vi "LVClasse_SurfaceFloat Set Data.vi"(0 "SurfaceFloat in":refnum<class "SurfaceFloat.lvclass">, 5 "data":sgl[][](array[numeric]), 11 "error in (no error)":errorcluster) -> (4 "SurfaceFloat out":refnum<class "SurfaceFloat.lvclass">, 15 "error out":errorcluster)   [LabVIEW 2020, in "SurfaceFloat.lvclass"]
doc: "Get write access Surface buffer.\n\n--------------------------------------------------------------------------------\n\n<B>SurfaceIn </B> : Surface object.\n<B>SurfaceOut </B> : Surface object.\n<B>data </B> : Surface buffer to set.\n<B>ErrorIn </B> : Error\n<B>ErrorOut </B> : Error\n\n--------------------------------------------------------------------------------"
uses:
  SurfaceFloat.lvclass
  SurfaceFloat.lvclass/SurfaceFloat.ctl
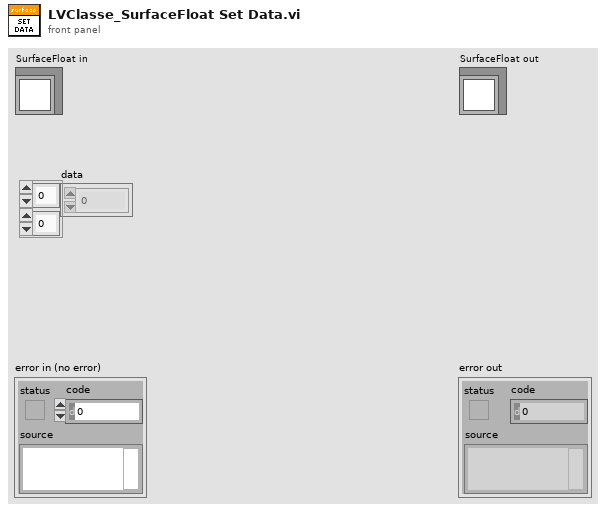
[diagram p1: front panel]
types:
  T1 = typedef "General dimensions definition.ctl" = cluster{"Size":T2, "Step":T3}
  T2 = typedef "Point2D.ctl" = cluster{"X":u32, "Y":u32}
  T3 = typedef "Point2Df.ctl" = cluster{"X":sgl, "Y":sgl}
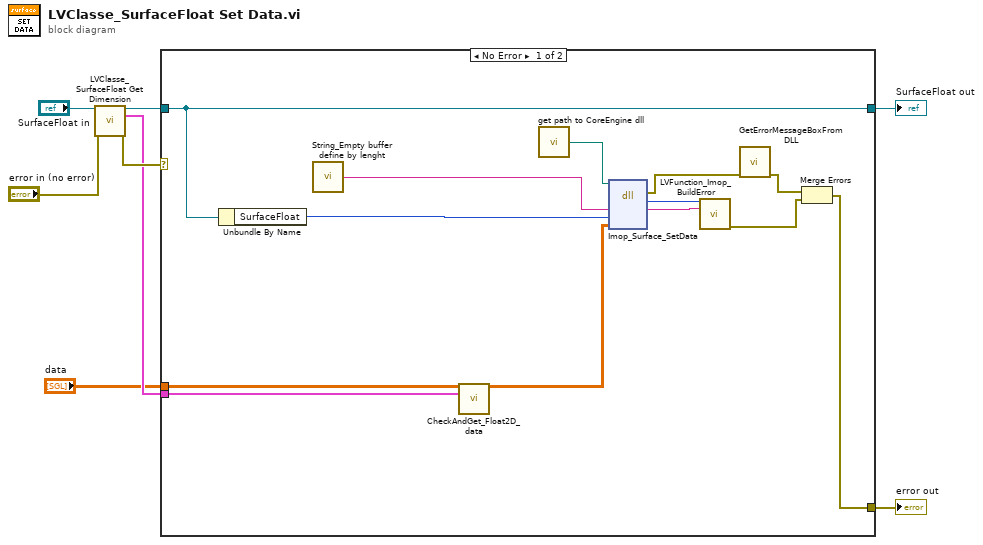
[diagram p0: block diagram]
diagram:
  n1 = call "LVClasse_SurfaceFloat Get Dimension.vi"("SurfaceFloat in"="SurfaceFloat in", "error in (no error)"="error in (no error)") -> ("SurfaceFloat out"=w3:refnum<class "SurfaceFloat.lvclass">, "Dimensions_um"=w2:T1, "error out"=w4:errorcluster)  [unwired: 11 in]
  n2 = case shown="No Error" w4 {
    selector: w4 -> [_ w23]
    tunnel: [w12 w23] -> w8
    tunnel: [w16 w22] -> w7
    tunnel: w3 -> [w16 w22]
    tunnel: w2 -> [w11 _]
    tunnel: "data" -> [w9 _]
    frame No Error {
      n3 = Unbundle By Name(w16) -> ("SurfaceFloat"=w15:i32)
      n4 = call "String_Empty buffer define by lenght.vi"() -> ("Empty buffer"=w19:string)  [unwired: 1 in]
      n5 = call "CheckAndGet_Float2D_data.vi"("data in"=w9, "Dimensions_um"=w11) -> ("data out"=w10:sgl[][])  [unwired: 13 in]
      n6 = call "get path to CoreEngine dll.vi"() -> ("path to c_interface_vc100.dll"=w18:path)  [unwired: 12 in, 3 out]
      n7 = dll-call lib="D:/2_trunk/Soft_haso/ImOpCoreEngine4_LV2011/DLLs/ImopEngine4_vc100.dll" fn="Imop_Surface_SetData"(path in=w18, "message"=w19, "surface"=w15, "data"=w10) -> (error out=w17:errorcluster, "return type"=w21:i32, "message"=w20:string)  [unwired: 4 in, 1 out]
      n8 = call "LVFunction_Imop_BuildError.vi"("code"=w21, "String to Prepend to source (\"\")"=w20) -> ("error out"=w13:errorcluster)  [unwired: 13 in]
      n9 = call "GetErrorMessageBoxFromDLL.vi"("error IN"=w17) -> ("error OUT"=w14:errorcluster)  [unwired: 10 in]
      n10 = Merge Errors(w14, w13) -> (w12:errorcluster)
    }
    frame Error {
    }
  }
  "error out" <- w8
  "SurfaceFloat out" <- w7
